vi "Set Dev Index wrapper.vi"(8 "error in (no error)":errorcluster caption="错误输入（无错误）", 10 "dwNewDevIndex":u32, 11 "dwPreDevIndex":u32) -> (0 "error out":errorcluster caption="错误输出", 3 "function return":u32)   [LabVIEW 2016, in "UISimCanFunc_wrapper.lvlib"]
doc: "_declspec (dllexport) DWORD SetDevIndex_wrapper(DWORD dwPreDevIndex, DWORD dwNewDevIndex);"
uses:
  <userlib>/UISimCanFunc_wrapper/UISimCanFunc_wrapper.lvlib
  <userlib>/UISimCanFunc_wrapper/UISimCanFunc_wrapper.dll
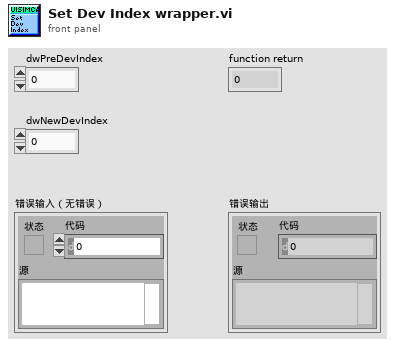
[diagram p1: front panel]
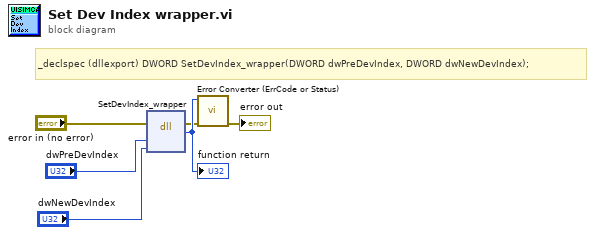
[diagram p0: block diagram]
diagram:
  # "_declspec (dllexport) DWORD SetDevIndex_wrapper(DWORD dwPreDevIndex, DWORD dwNewDevIndex);"
  n1 = dll-call lib="C:/Program Files (x86)/National Instruments/LabVIEW 2016/user.lib/UISimCanFunc_wrapper/UISimCanFunc_wrapper.*" fn="SetDevIndex_wrapper"(error in="error in (no error)", "dwPreDevIndex"="dwPreDevIndex", "dwNewDevIndex"="dwNewDevIndex") -> (error out=w2:errorcluster, w6:u32)  [unwired: 4 in, 1 out]
  "function return" <- w6
  n2 = call <userlib>:"Error Converter (ErrCode or Status).vi"("error in (no error)"=w2, "error code"=w6) -> ("error out"=→"error out":errorcluster)  [unwired: 9 in]
